vi "W Command.vi"(8 "error in (no error)":errorcluster, 11 "PSP-405 resource in":refnum<visa-resource-name>) -> (0 "error out":errorcluster, 2 "power value":dbl, 3 "PSP-405 resource out":refnum<visa-resource-name>, 4 "raw response":string)   [LabVIEW 2017, in "GW Instek PSP-405.lvlib"]
doc: "The W query returns the load output of the power supply."
uses:
  GW Instek PSP-405.lvlib
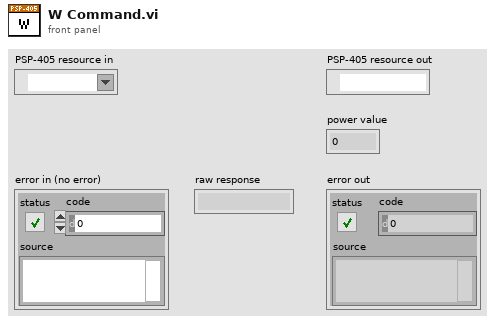
[diagram p1: front panel]
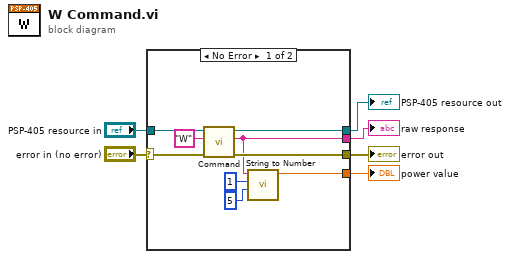
[diagram p0: block diagram]
diagram:
  n1 = case shown="No Error" "error in (no error)" {
    selector: "error in (no error)" -> [w12 w17]
    tunnel: "PSP-405 resource in" -> [w14 w16]
    tunnel: [w10 _] -> w5
    tunnel: [w15 w17] -> w4
    tunnel: [w11 w16] -> w2
    tunnel: [w7 _] -> w1
    frame No Error {
      n2 = call "Command.vi"("error in (no error)"=w12, "cmd"="W", "PSP-405 resource in"=w14) -> ("error out"=w15:errorcluster, "response"=w10:string, "PSP-405 resource out"=w11:refnum<visa-resource-name>)  [unwired: 6 in]
      n3 = call "String to Number.vi"("length"=5, "offset"=1, "string"=w10) -> ("numeric"=w7:dbl)  [unwired: 8 in]
    }
    frame Error {
    }
  }
  "error out" <- w4
  "raw response" <- w5
  "PSP-405 resource out" <- w2
  "power value" <- w1
